vi "ExSetup2stripbc.vi"() -> ()   [LabVIEW 2010]
uses:
  Open-Close Hardware/CamHandle.vi
panel:
  out "bit depth":i32
  out "Readout Port":i32
  out "Pixel time":i32
  out "Gain":i32
  in  "ADC gain":i32=-1
  in  "ADC port":i32=3
  in  "ADC speed":i32=-3
  out "ADC Speed":u32
  out "error out":errorcluster
  in  "error in (no error)":errorcluster
  in  "Timing Mode":u32(ring)=1 items=["N/A", "Timed Mode/Free run", "Trigger First (only PM)", "Strobed/Ext Sync", "Bulb Mode (PM only)", "Variable Timed mode (PM only)", "Flash Mode (only some PM)"]
  in  "x1":u32=1
  in  "x2":u32=500
  in  "y1":u32
  in  "y2":u32=49
  in  "x bin":u32=1
  in  "y bin":u32=25
  in  "x1 s2":u32=1
  in  "x2 s2":u32=500
  in  "y1 s2":u32=26
  in  "y2 s2":u32=50
  in  "x bin s2":u32=1
  in  "y bin s2":u32=25
  in  "min block":u32=2
  in  "Num Min Block":u32=5
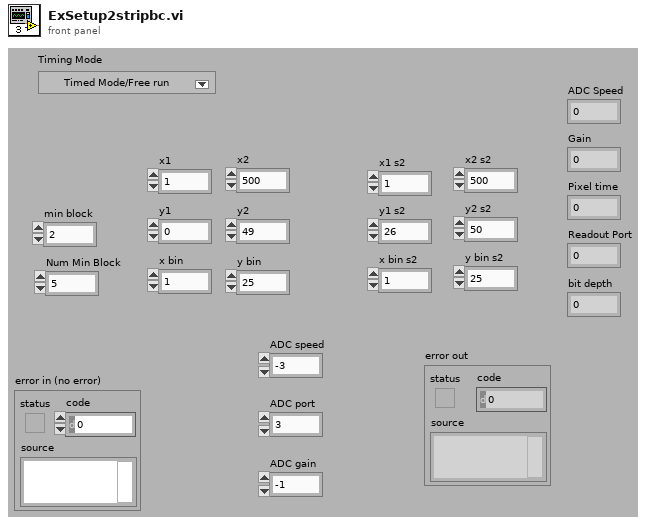
[diagram p1: front panel]
types:
  T1 = cluster{"x1":u32, "x2":u32, "x bin":u32, "y1":u32, "y2":u32, "y bin":u32}
  T2 = cluster{"x1 s2":u32, "x2 s2":u32, "x bin s2":u32, "y1 s2":u32, "y2 s2":u32, "y bin s2":u32}
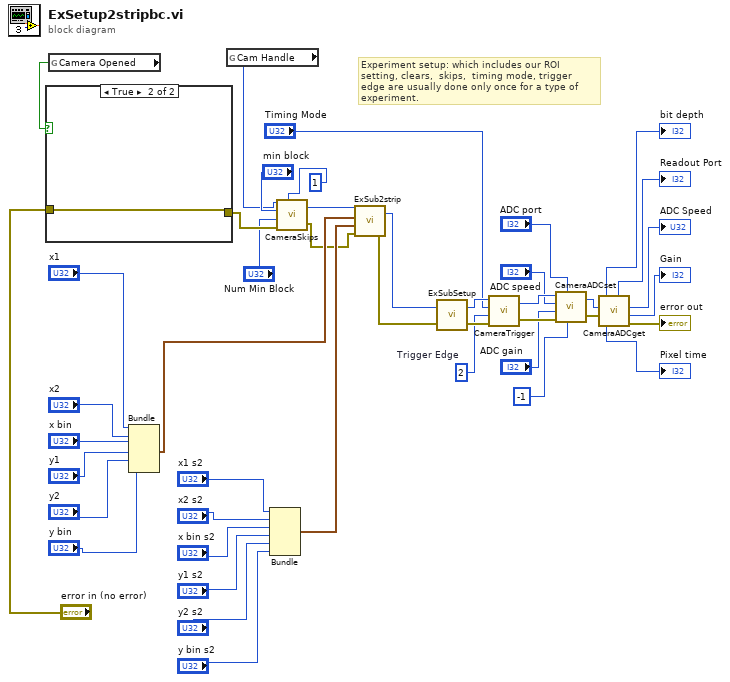
[diagram p0: block diagram]
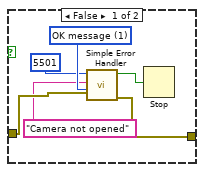
[diagram p2: hidden frame]
diagram:
  w41 = u32 2  # Trigger Edge
  # "Experiment setup: which includes our ROI setting, clears,  skips,  timing mode, trigger edge are usually done only once for a type of experiment."
  n1 = global read "CamHandle.vi" "Camera Opened"() -> (w40:bool)
  n2 = case shown="True" w40 {
    tunnel: "error in (no error)" -> [w48 w50]
    tunnel: [w47 w50] -> w21
    frame False {
      w49 = u16 1 items=["no dialog", "OK message", "continue or stop message"] ("type of dialog (OK msg:1)")
      n3 = call <vilib>:"Simple Error Handler.vi"("error code (no error:0)"=5501, "error source (\" \")"="Camera not opened", "type of dialog (OK msg:1)"=w49, "error in (no error)"=w48) -> ("error?"=w45:bool, "error out"=w47:errorcluster)  [unwired: 1 in, 3 out]
      n4 = Stop(stop? (T)=w45) -> ()
    }
    frame True {
    }
  }
  n5 = Bundle("x1"="x1", "x2"="x2", "x bin"="x bin", "y1"="y1", "y2"="y2", "y bin"="y bin") -> (w29:T1)  [unwired: 1 in]
  n6 = global read "CamHandle.vi" "Cam Handle"() -> (w14:u32)
  n7 = Bundle("x1 s2"="x1 s2", "x2 s2"="x2 s2", "x bin s2"="x bin s2", "y1 s2"="y1 s2", "y2 s2"="y2 s2", "y bin s2"="y bin s2") -> (w22:T2)  [unwired: 1 in]
  n8 = call <userlib>:"CameraSkips.vi"("Camera Handle"=w14, "Minimum Block Size"="min block", "Number of Minimum blocks"="Num Min Block", "error in"=w21, "Type of Skips"=1) -> ("Camera Handle"=w19:u32, "error out"=w20:errorcluster)
  n9 = call "ExSub2strip.vi"("error in (no error)"=w20, "strip 2"=w22, "strip 1"=w29, "Camera Handle"=w19) -> ("error out"=w36:errorcluster, "Camera Handle"=w15:u32)
  n10 = call "ExSubSetup.vi"("error in (no error)"=w36, "Camera Handle"=w15) -> ("error out"=w42:errorcluster, "Camera Handle"=w43:u32)
  n11 = call <userlib>:"CameraTrigger.vi"("error in"=w42, "Trigger Edge"=w41, "Timing Mode"="Timing Mode", "Camera Handle"=w43) -> ("error out"=w39:errorcluster, "Camera Handle"=w38:u32)
  n12 = call <userlib>:"CameraADCset.vi"("ADC offset"=-1, "Read Out port"="ADC port", "error in (no error)"=w39, "ADC Gain"="ADC gain", "ADC Speed"="ADC speed", "Camera Handle"=w38) -> ("error out"=w11:errorcluster, "Camera Handle"=w5:u32)
  n13 = call <userlib>:"CameraADCget.vi"("Camera handle"=w5, "error in (no error)"=w11) -> ("Bit Depth"=→"bit depth":i32, "Pixel Time"=→"Pixel time":i32, "Readout Port"=→"Readout Port":i32, "ADC Speed"=→"ADC Speed":i32, "ADC Gain"=→"Gain":i32, "error out"=→"error out":errorcluster)  [unwired: 2 out]
